vi "get channels.vi"(11 "fixed channel configuration in":refnum<class "control module configuration.lvclass">) -> (2 "channels":refnum<class "TBM channel.lvclass">[](array[class]), 3 "fixed channel configuration out":refnum<class "control module configuration.lvclass">)   [LabVIEW 2013, in "control module configuration.lvclass"]
uses:
  control module configuration.lvclass
  <vilib>/NI/Tag Bus Module Framework/channel/TBM channel.lvclass
  control module configuration.lvclass/control module configuration.ctl
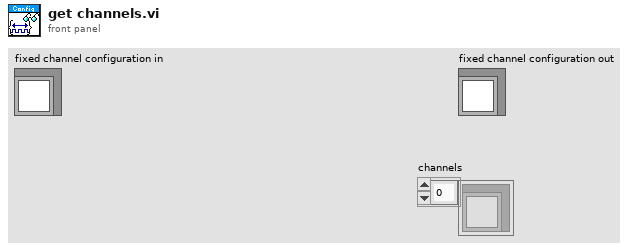
[diagram p1: front panel]
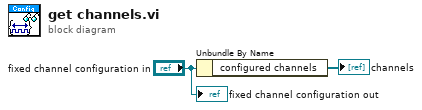
[diagram p0: block diagram]
diagram:
  n1 = Unbundle By Name("fixed channel configuration in") -> ("configured channels"=→"channels":refnum<class "TBM channel.lvclass">[])
  "fixed channel configuration out" <- "fixed channel configuration in"
